vi "Deploy Via.vi"(8 "error in (no error)":errorcluster, 10 "VIA":string, 11 "Device in":refnum<class "Device.lvclass">) -> (0 "error out":errorcluster, 2 "Response":string, 3 "Device out":refnum<class "Device.lvclass">)   [LabVIEW 2020, in "PicoG-Core.lvlib" / "Device.lvclass"]
uses:
  Device.lvclass
  Device.lvclass/Device.ctl
  DeployPlatform/DeployPlatform.lvclass
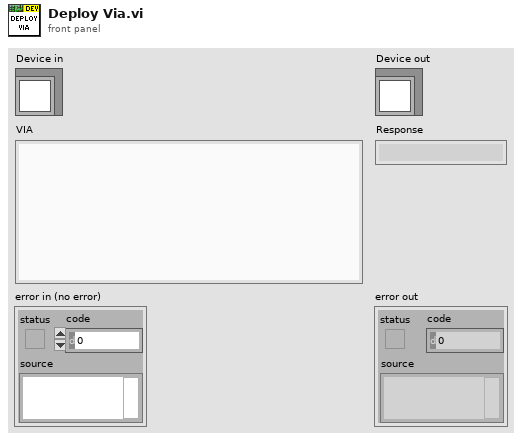
[diagram p1: front panel]
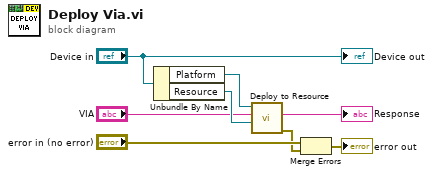
[diagram p0: block diagram]
diagram:
  n1 = Unbundle By Name("Device in") -> ("Platform"=w6:refnum<class "DeployPlatform.lvclass">, "Resource"=w5:refnum<class "DeployResource.lvclass">)
  n2 = call-dynamic "Deploy to Resource.vi"("Resource"=w5, "VIA"="VIA", "DeployTarget in"=w6) -> ("error out"=w1:errorcluster, "Response"=→"Response":string)  [unwired: 6 in, 1 out]
  n3 = Merge Errors("error in (no error)", w1) -> (→"error out":errorcluster)
  "Device out" <- "Device in"
